vi "Run Sample Metadata.vi"(0 "Image File (Path/Name)":path) -> ()   [LabVIEW 2016]
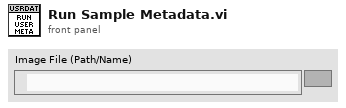
[diagram p1: front panel]
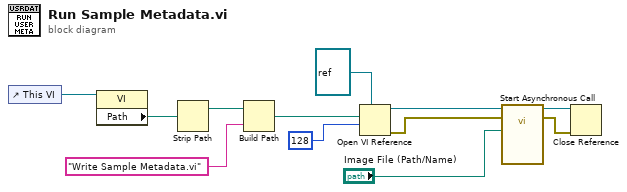
[diagram p0: block diagram]
diagram:
  n1 = control-ref of="This VI"() -> (w12:refnum<vi>)
  n2 = property class="VI"(reference=w12) -> ("Path"=w11:path)  [unwired: 1 in, 2 out]
  n3 = Strip Path(path=w11) -> (stripped path=w10:path)  [unwired: 1 out]
  n4 = Build Path(base path=w10, name or relative path="Write Sample Metadata.vi") -> (appended path=w8:path)
  n5 = Open VI Reference(type specifier VI Refnum (for type only)=refnum<vi> refnum, vi path=w8, options=128) -> (vi reference=w5:refnum<vi>, error out=w3:errorcluster)  [unwired: 3 in]
  n6 = call-by-ref "Start Asynchronous Call"(reference=w5, error in=w3, "File Path"="Image File (Path/Name)") -> (reference out=w4:refnum<vi>, error out=w2:errorcluster)  [unwired: 12 in, 3 out]
  n7 = Close Reference(reference=w4, error in (no error)=w2) -> ()  [unwired: 1 out]
